vi "Event Handler.vi"(0 "Kasli Wrapper in":refnum<class "Kasli Wrapper 2.0.lvclass">, 5 "Event type":T1=enum."Message", 7 "Item Name":string, 9 "Data":variant, 11 "error in (no error)":errorcluster) -> (4 "Kasli Wrapper out":refnum<class "Kasli Wrapper 2.0.lvclass">, 15 "error out":errorcluster)   [LabVIEW 2020, in "Kasli Wrapper 2.0.lvlib" / "Kasli Wrapper 2.0.lvclass"]
doc: "This VI is the event handler of the uService: every time an event is triggered to the uService, this VI is called.\nNote: here you can access the Actor/Class data, but it will be the one coming out from Init. You cannot modify the values.\nThree different events are supported:\nI) Button Pressed: get called on a GUI button pressed. Item Name is the name (label) of the button, Data is empty.\nII) Shared Variable Updated: get called when a SV you subscribed to is updated. Item Name is the name of the SV, and Data is the value (note: you need to convert it to the proper type).\nIII) Message: get called every time a user event is generated using Send Message to Event Handler. The values of Item Name and Data are the one given to the Send Message to Event Handler.\nIV) Ready to launch?: this frame get called every time a new Run is initiated. Each uService is responsible of performing a self check before giving back the green light for the Run to start."
uses:
  Kasli Wrapper 2.0.lvclass
  C:/Users/aegis/Documents/CIRCUS/TALOS/TALOS_PPL.lvlibp/Father of all uServices/Father of all uServices/Father of all uServices.lvclass
  TALOS/TALOS_PPL.lvlibp/Father of all uServices/Father of all uServices/Event Handler Items.ctl
  Kasli Wrapper 2.0 Consumer Case Selector.ctl
  Run Utilities/TypeDefs/Messages/Submit Message.ctl
  Run Utilities/TypeDefs/DAQ Control.ctl
  Run Utilities/Run Instance/Run Instance.lvclass
  Kasli Wrapper 2.0.lvclass/Kasli Wrapper 2.0.ctl
  TALOS/TALOS_PPL.lvlibp/Father of all uServices/Father of all uServices/Father of all uServices.lvclass
  Run Utilities/Run Utilities.lvlib
  TALOS/TALOS_PPL.lvlibp
  C:/Users/aegis/Documents/CIRCUS/TALOS/TALOS_PPL.lvlibp/Ancestor/Ancestor/Ancestor.lvclass
  C:/Users/aegis/Documents/CIRCUS/TALOS/Actor Framework.lvlibp/1abvi3w/vi.lib/ActorFramework/Actor/Actor.lvclass
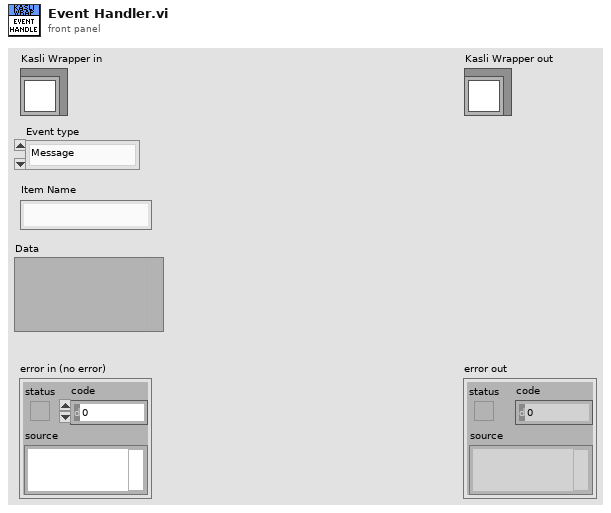
[diagram p1: front panel]
types:
  T1 = typedef "TALOS_PPL.lvlibp/Father of all uServices.lvlib/Father of all uServices.lvclass/Event Handler Items.ctl" = enum16{"Button Pressed", "Shared Variable Updated", "Message", "Ready to launch?", "Safe Mode", "Start RUN", "Stop RUN"}
  T2 = typedef "Kasli Wrapper 2.0.lvlib/Kasli Wrapper 2.0.lvclass/Kasli Wrapper 2.0 Consumer Case Selector.ctl" = enum16{"Init", "Submit Script", "Restart Master", "Master StdOut", "Master StdErr", "Client StdOut", "Client StdErr", "Start Logging", "Stop Logging", "Terminate Script", "Close", "Master ProcessExit"}
  T3 = typedef "Run Utilities.lvlib/DAQ Control.ctl" = enum16{"On", "Off", "External"}
  T4 = typedef "Run Utilities.lvlib/Submit Message.ctl" = cluster{"DAQ Control":T3, "Run Instance":refnum<class "Run Instance.lvclass">}
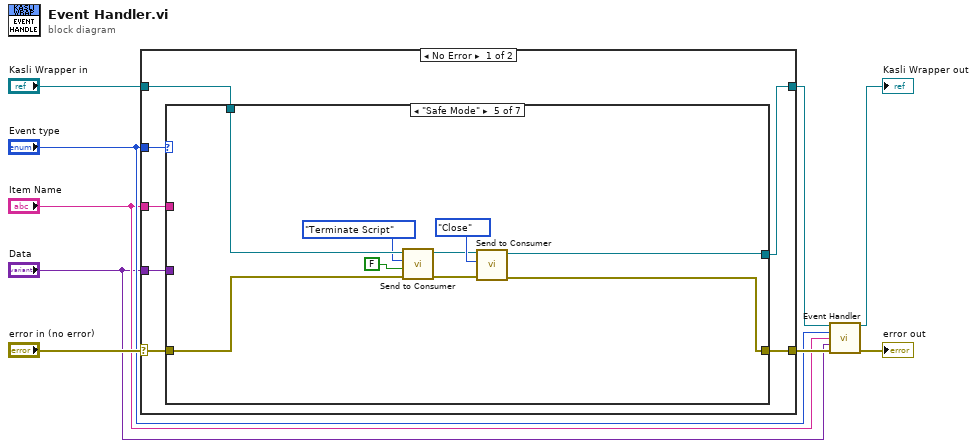
[diagram p0: block diagram]
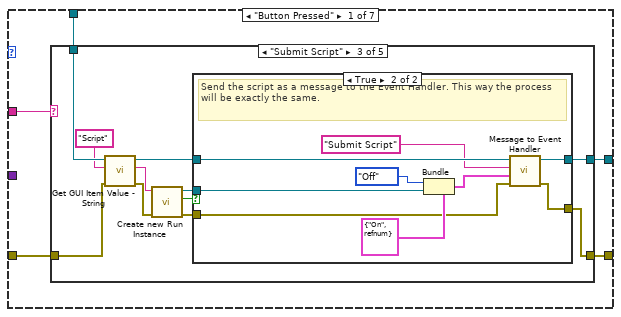
[diagram p2: hidden frame]
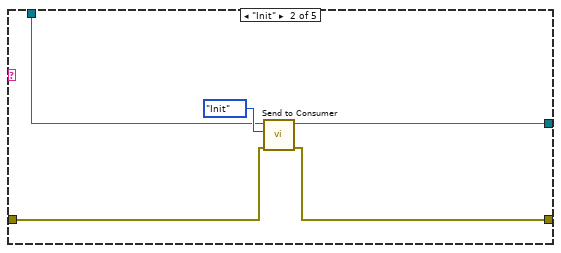
[diagram p4: hidden frame]
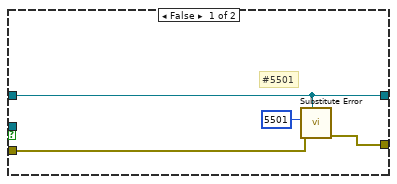
[diagram p5: hidden frame]
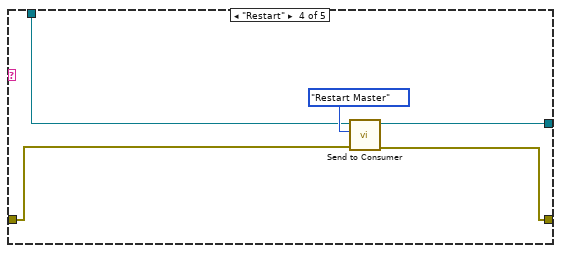
[diagram p6: hidden frame]
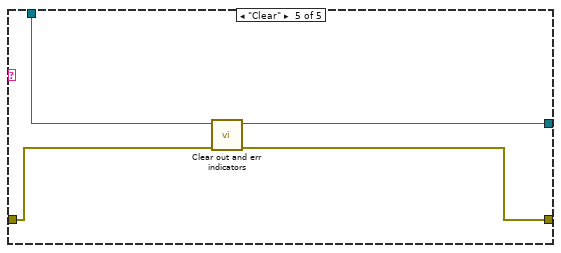
[diagram p7: hidden frame]
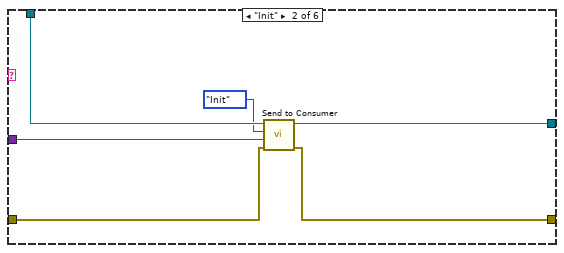
[diagram p10: hidden frame]
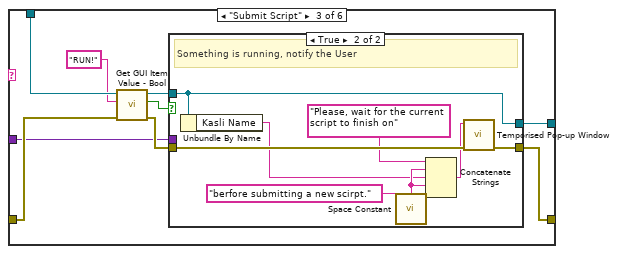
[diagram p11: hidden frame]
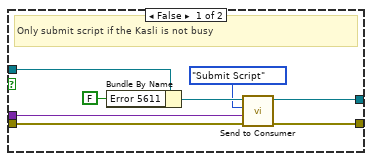
[diagram p12: hidden frame]
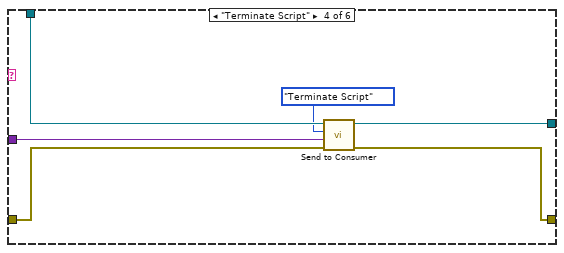
[diagram p13: hidden frame]
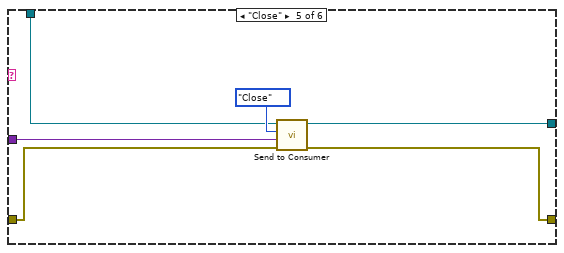
[diagram p14: hidden frame]
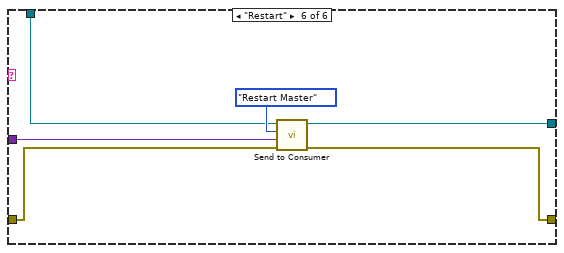
[diagram p15: hidden frame]
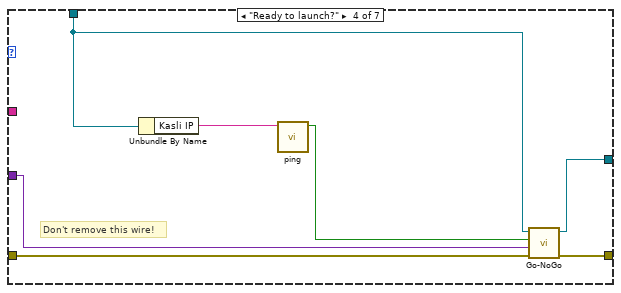
[diagram p16: hidden frame]
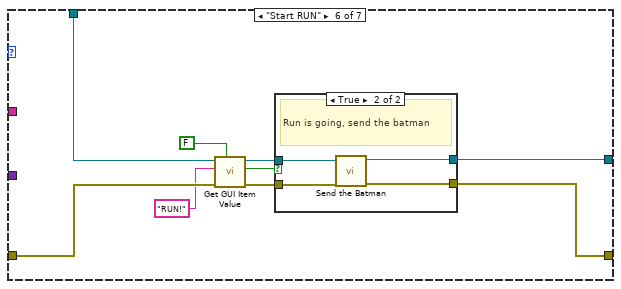
[diagram p17: hidden frame]
diagram:
  n1 = case shown="No Error" "error in (no error)" {
    selector: "error in (no error)" -> [w14 w155]
    tunnel: [w15 w155] -> w7
    tunnel: [w10 w154] -> w4
    tunnel: "Kasli Wrapper in" -> [w13 w154]
    tunnel: "Event type" -> [w16 _]
    tunnel: "Item Name" -> [w12 _]
    tunnel: "Data" -> [w11 _]
    frame No Error {
      n2 = case shown="\"Safe Mode\"" w16 {
        tunnel: [w18 w63 w65 w127 w134 w144 w152] -> w15
        tunnel: w14 -> [w19 w63 w69 w124 w130 w138 w152]
        tunnel: w12 -> [w20 _ w68 _ _ _ _]
        tunnel: w13 -> [w21 w62 w66 w122 w133 w140 w153]
        tunnel: w11 -> [_ _ w67 w126 _ _ _]
        tunnel: [w17 w62 w64 w121 w135 w145 w153] -> w10
        frame "Button Pressed" {
          n3 = case shown="\"Submit Script\"" w20 {
            tunnel: w19 -> [w23 w27 w36 w54 w60]
            tunnel: w21 -> [w22 w24 w37 w53 w61]
            tunnel: [w23 w26 w39 w56 w58] -> w18
            tunnel: [w22 w25 w29 w55 w59] -> w17
            frame Default {
            }
            frame "Init" {
              n4 = call "Send to Consumer.vi"("error in (no error)"=w27, "Case ID"=Kasli_Wrapper_2.0_Consumer_Case_Selector."Init" ("Consumer Case Selector"), "uService Template in"=w24) -> ("error out"=w26:errorcluster, "uService Template out"=w25:refnum<class "Kasli Wrapper 2.0.lvclass">)  [unwired: 7 in]
            }
            frame "Submit Script" {
              n5 = call "Get GUI Item Value - String.vi"("error in (no error)"=w36, "FP Item Name"="Script", "uService Template in"=w37) -> ("error out"=w33:errorcluster, "Value"=w30:string, "uService Template out"=w38:refnum<class "Kasli Wrapper 2.0.lvclass">)  [unwired: 6 in]
              n6 = call "Create new Run Instance.vi"("error in"=w33, "Script Name"=w30) -> ("error out"=w34:errorcluster, "Created?"=w31:bool, "Run Instance"=w32:refnum<class "Run Instance.lvclass">)  [unwired: 7 in]
              n7 = case shown="True" w31 {
                tunnel: [w42 w47] -> w39
                tunnel: w38 -> [w40 w49]
                tunnel: w34 -> [w43 w46]
                tunnel: w32 -> [_ w51]
                tunnel: [w40 w48] -> w29
                frame False {
                  # "#5501"
                  n8 = call "Substitute Error.vi"("LabVIEW Object"=w40, "error in (no error)"=w43, "Error Code"=5501) -> ("error out"=w42:errorcluster)  [unwired: 8 in]
                }
                frame True {
                  # "Send the script as a message to the Event Handler. This way the process will be exactly the same."
                  n9 = Bundle(cluster=T4 {"DAQ Control"=enum."On", "Run Instance"=refnum} ("Submit Msg"), "DAQ Control"=DAQ_Control."Off", "Run Instance"=w51) -> (w45:T4)
                  n10 = call "Message to Event Handler.vi"("error in (no error)"=w46, "Data"=w45, "Item Name"="Submit Script", "uService Template in"=w49) -> ("error out"=w47:errorcluster, "uService Template out"=w48:refnum<class "Kasli Wrapper 2.0.lvclass">)  [unwired: 6 in]
                }
              }
            }
            frame "Restart" {
              n11 = call "Send to Consumer.vi"("error in (no error)"=w54, "Case ID"=Kasli_Wrapper_2.0_Consumer_Case_Selector."Restart Master" ("Consumer Case Selector"), "uService Template in"=w53) -> ("error out"=w56:errorcluster, "uService Template out"=w55:refnum<class "Kasli Wrapper 2.0.lvclass">)  [unwired: 7 in]
            }
            frame "Clear" {
              n12 = call-dynamic "Clear out and err indicators.vi"("error in (no error)"=w60, "Kasli Wrapper 2.0 in"=w61) -> ("error out"=w58:errorcluster, "Kasli Wrapper 2.0 out"=w59:refnum<class "Kasli Wrapper 2.0.lvclass">)  [unwired: 8 in]
            }
          }
        }
        frame "Shared Variable Updated" {
        }
        frame "Message" {
          n13 = case shown="Default" w68 {
            tunnel: w69 -> [w71 w74 w86 w105 w111 w117]
            tunnel: w67 -> [_ w75 w84 w104 w113 w119]
            tunnel: w66 -> [w70 w77 w79 w108 w112 w118]
            tunnel: [w71 w73 w83 w106 w110 w116] -> w65
            tunnel: [w70 w72 w82 w107 w109 w115] -> w64
            frame Default {
            }
            frame "Init" {
              n14 = call "Send to Consumer.vi"("error in (no error)"=w74, "Data"=w75, "Case ID"=Kasli_Wrapper_2.0_Consumer_Case_Selector."Init" ("Consumer Case Selector"), "uService Template in"=w77) -> ("error out"=w73:errorcluster, "uService Template out"=w72:refnum<class "Kasli Wrapper 2.0.lvclass">)  [unwired: 6 in]
            }
            frame "Submit Script" {
              n15 = call "Get GUI Item Value - Bool.vi"("error in (no error)"=w86, "FP Item Name"="RUN!", "uService Template in"=w79) -> ("error out"=w85:errorcluster, "Value"=w80:bool, "uService Template out"=w81:refnum<class "Kasli Wrapper 2.0.lvclass">)  [unwired: 6 in]
              n16 = case shown="True" w80 {
                tunnel: w85 -> [w94 w102]
                tunnel: w84 -> [w91 _]
                tunnel: [w90 w101] -> w83
                tunnel: [w88 w98] -> w82
                tunnel: w81 -> [w87 w98]
                frame False {
                  # "Only submit script if the Kasli is not busy"
                  n17 = Bundle By Name(cluster=w87, "Error 5611"=FALSE ("Error 6666")) -> (w93:refnum<class "Kasli Wrapper 2.0.lvclass">)
                  n18 = call "Send to Consumer.vi"("error in (no error)"=w94, "Data"=w91, "Case ID"=Kasli_Wrapper_2.0_Consumer_Case_Selector."Submit Script" ("Consumer Case Selector"), "uService Template in"=w93) -> ("error out"=w90:errorcluster, "uService Template out"=w88:refnum<class "Kasli Wrapper 2.0.lvclass">)  [unwired: 6 in]
                }
                frame True {
                  # "Something is running, notify the User"
                  n19 = Unbundle By Name(w98) -> ("Kasli Name"=w96:string)
                  n20 = call <vilib>:"Space Constant.vi"() -> ("String"=w97:string)
                  n21 = Concatenate Strings("Please, wait for the current script to finish on" ("Text"), w97, w96, w97, "berfore submitting a new scirpt." ("string")) -> (w99:string)
                  n22 = call "Temporised Pop-up Window.vi"("error in (no error)"=w102, "Text"=w99) -> ("error out"=w101:errorcluster)  [unwired: 9 in]
                }
              }
            }
            frame "Terminate Script" {
              n23 = call "Send to Consumer.vi"("error in (no error)"=w105, "Data"=w104, "Case ID"=Kasli_Wrapper_2.0_Consumer_Case_Selector."Terminate Script" ("Consumer Case Selector"), "uService Template in"=w108) -> ("error out"=w106:errorcluster, "uService Template out"=w107:refnum<class "Kasli Wrapper 2.0.lvclass">)  [unwired: 6 in]
            }
            frame "Close" {
              n24 = call "Send to Consumer.vi"("error in (no error)"=w111, "Data"=w113, "Case ID"=Kasli_Wrapper_2.0_Consumer_Case_Selector."Close" ("Consumer Case Selector"), "uService Template in"=w112) -> ("error out"=w110:errorcluster, "uService Template out"=w109:refnum<class "Kasli Wrapper 2.0.lvclass">)  [unwired: 6 in]
            }
            frame "Restart" {
              n25 = call "Send to Consumer.vi"("error in (no error)"=w117, "Data"=w119, "Case ID"=Kasli_Wrapper_2.0_Consumer_Case_Selector."Restart Master" ("Consumer Case Selector"), "uService Template in"=w118) -> ("error out"=w116:errorcluster, "uService Template out"=w115:refnum<class "Kasli Wrapper 2.0.lvclass">)  [unwired: 6 in]
            }
          }
        }
        frame "Ready to launch?" {
          # "Don't remove this wire!"
          n26 = Unbundle By Name(w122) -> ("Kasli IP"=w125:string)
          n27 = call "ping.vi"("IP/Address"=w125) -> ("Success?"=w123:bool)  [unwired: 7 in, 3 out]
          n28 = call-dynamic "Go-NoGo.vi"("error in (no error)"=w124, "Go-NoGo Data"=w126, "Go?"=w123, "Father of all uServices in"=w122) -> ("error out"=w127:errorcluster, "Father of all uServices out"=w121:refnum<class "Kasli Wrapper 2.0.lvclass">)  [unwired: 6 in]
        }
        frame "Safe Mode" {
          n29 = call "Send to Consumer.vi"("error in (no error)"=w130, "Data"=FALSE, "Case ID"=Kasli_Wrapper_2.0_Consumer_Case_Selector."Terminate Script" ("Consumer Case Selector"), "uService Template in"=w133) -> ("error out"=w131:errorcluster, "uService Template out"=w132:refnum<class "Kasli Wrapper 2.0.lvclass">)  [unwired: 6 in]
          n30 = call "Send to Consumer.vi"("error in (no error)"=w131, "Case ID"=Kasli_Wrapper_2.0_Consumer_Case_Selector."Close" ("Consumer Case Selector"), "uService Template in"=w132) -> ("error out"=w134:errorcluster, "uService Template out"=w135:refnum<class "Kasli Wrapper 2.0.lvclass">)  [unwired: 7 in]
        }
        frame "Start RUN" {
          n31 = call-poly "Get GUI Item Value.vi"("Default"=FALSE, "error in (no error)"=w138, "FP Item Name"="RUN!", "uService Template in"=w140) -> ("error out"=w139:errorcluster, "Value"=w142:bool, "uService Template out"=w141:refnum<class "Kasli Wrapper 2.0.lvclass">)  [unwired: 5 in]
          n32 = case shown="True" w142 {
            tunnel: [w146 w151] -> w145
            tunnel: [w147 w150] -> w144
            tunnel: w141 -> [w146 w149]
            tunnel: w139 -> [w147 w148]
            frame False {
            }
            frame True {
              # "Run is going, send the batman"
              n33 = call-dynamic "Send the Batman.vi"("error in (no error)"=w148, "Kasli Wrapper 2.0 in"=w149) -> ("error out"=w150:errorcluster, "Kasli Wrapper 2.0 out"=w151:refnum<class "Kasli Wrapper 2.0.lvclass">)  [unwired: 8 in]
            }
          }
        }
        frame "Stop RUN" {
        }
      }
    }
    frame Error {
    }
  }
  n34 = call-parent "Event Handler.vi"("uService Template in"=w4, "Event type"="Event type", "Item Name"="Item Name", "Data"="Data", "error in (no error)"=w7) -> ("uService Template out"=→"Kasli Wrapper out":refnum<class "Kasli Wrapper 2.0.lvclass">, "error out"=→"error out":errorcluster)  [unwired: 9 in]
